vi "Set Baud Rate.vi"(8 "error in":errorcluster, 10 "Baud Rate":u32, 11 "IHas Baudrate in":refnum<class "IHas Baud Rate.lvclass">) -> (0 "error out":errorcluster, 3 "IHas Baudrate out":refnum<class "IHas Baud Rate.lvclass">)   [LabVIEW 2024, in "IHas Baud Rate.lvclass"]
uses:
  IHas Baud Rate.lvclass
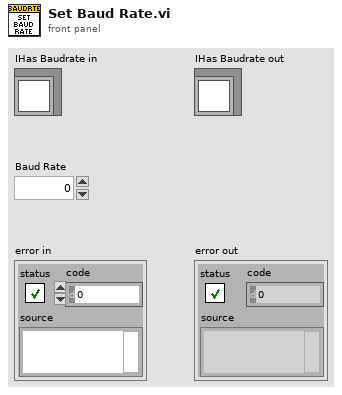
[diagram p1: front panel]
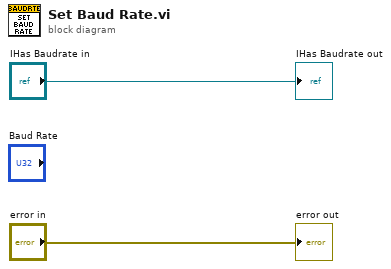
[diagram p0: block diagram]
diagram:
  "error out" <- "error in"
  "IHas Baudrate out" <- "IHas Baudrate in"
